vi "WristExecute.vi"(8 "error in (no error)":errorcluster) -> (0 "error out":errorcluster)   [LabVIEW 2023]
uses:
  <vilib>/Rock Robotics/WPI/ThirdParty/JAS_Junk/TrajLib/Trajectory_Library.lvlib
  WristGlobal.vi
  <vilib>/Rock Robotics/WPI/ThirdParty/REV Robotics/REVLib/SubVI/Public/SPARK Get Encoder Status Position.vi
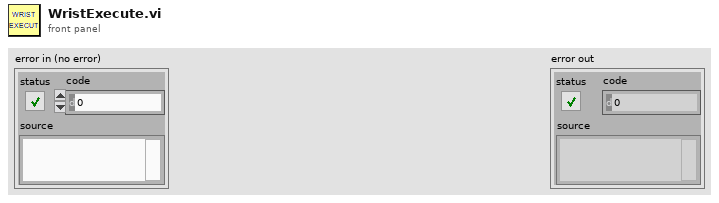
[diagram p1: front panel]
types:
  T1 = typedef "WPI_MotorControlDeviceRef.ctl" = cluster{"DeviceStatus":errorcluster, "Type":T2, "PWM":cluster{"PWM Channel":T3, "DeadBand":T4}, "CAN":cluster{"Device Number":u8, "SetOutput VI Ref":variant, "GetOutput VI Ref":variant, "Enable VI Ref":variant, "Disable VI Ref":variant, "Data":variant}, "Invert":bool, "DIO PWM":cluster{"PWM \"Enable\" Channel":T3, "DIOChannel":T5, "PWM Rate":dbl}}
  T2 = typedef "WPI_MotorControlType.ctl" = enum16{"PWM", "CAN", "DIO PWM"}
  T3 = typedef "FPGA_DIOPWMChannel.ctl" = enum8{"PWM 0", "PWM 1", "PWM 2", "PWM 3", "PWM 4", "PWM 5", "PWM 6", "PWM 7", "PWM 8", "PWM 9", "PWM MXP 0", "PWM MXP 1", "PWM MXP 2", "PWM MXP 3", "PWM MXP 4", "PWM MXP 5", "PWM MXP 6", "PWM MXP 7", "PWM MXP 8", "PWM MXP 9", "Invalid"}
  T4 = typedef "WPI_PWMDeadband.ctl" = cluster{"Name":string, "maxPositivePwm":i32, "minPositivePwm":i32, "centerPwm":i32, "maxNegativePwm":i32, "minNegativePwm":i32, "angularRange":u16}
  T5 = typedef "FPGA_DIOChannel.ctl" = enum8{"DIO 0", "DIO 1", "DIO 2", "DIO 3", "DIO 4", "DIO 5", "DIO 6", "DIO 7", "DIO 8", "DIO 9", "DIO MXP 0", "DIO MXP 1", "DIO MXP 2", "DIO MXP 3", "DIO MXP 4", "DIO MXP 5", "DIO MXP 6", "DIO MXP 7", "DIO MXP 8", "DIO MXP 9", "DIO MXP 10", "DIO MXP 11", "DIO MXP 12", "DIO MXP 13", "DIO MXP 14", "DIO MXP 15", "SPI Port CS1", "SPI Port CS2", "SPI Port CS3", "SPI Port MISO", "SPI Port MOSI", "Invalid"}
  T6 = typedef "WPI_EncoderDevRef.ctl" = cluster{"DevStatus":errorcluster, "EncoderIndex":T7, "CounterIndex":T8, "DistancePerCount":dbl, "Decoding Type":T9}
  T7 = typedef "FPGA_EncoderIdx.ctl" = enum8{"Enc 0", "Enc 1", "Enc 2", "Enc 3", "Enc 4", "Enc 5", "Enc 6", "Enc 7", "Invalid"}
  T8 = typedef "FPGA_CounterCtrSystemIndex.ctl" = enum8{"Ctr 0", "Ctr 1", "Ctr 2", "Ctr 3", "Ctr 4", "Ctr 5", "Ctr 6", "Ctr 7", "Invalid"}
  T9 = typedef "WPI_EncoderType.ctl" = enum16{"1x", "2x", "4x"}
  T10 = typedef "Trajectory_Library.lvlib/PosCtrl_Tuning_Type.ctl" = cluster{"Slope":dbl, "Offset":dbl, "Error Deadband":dbl, "At Reference Count":i32, "Negate Output":bool, "Max Allowd Position":dbl, "Min Allowd Position":dbl}
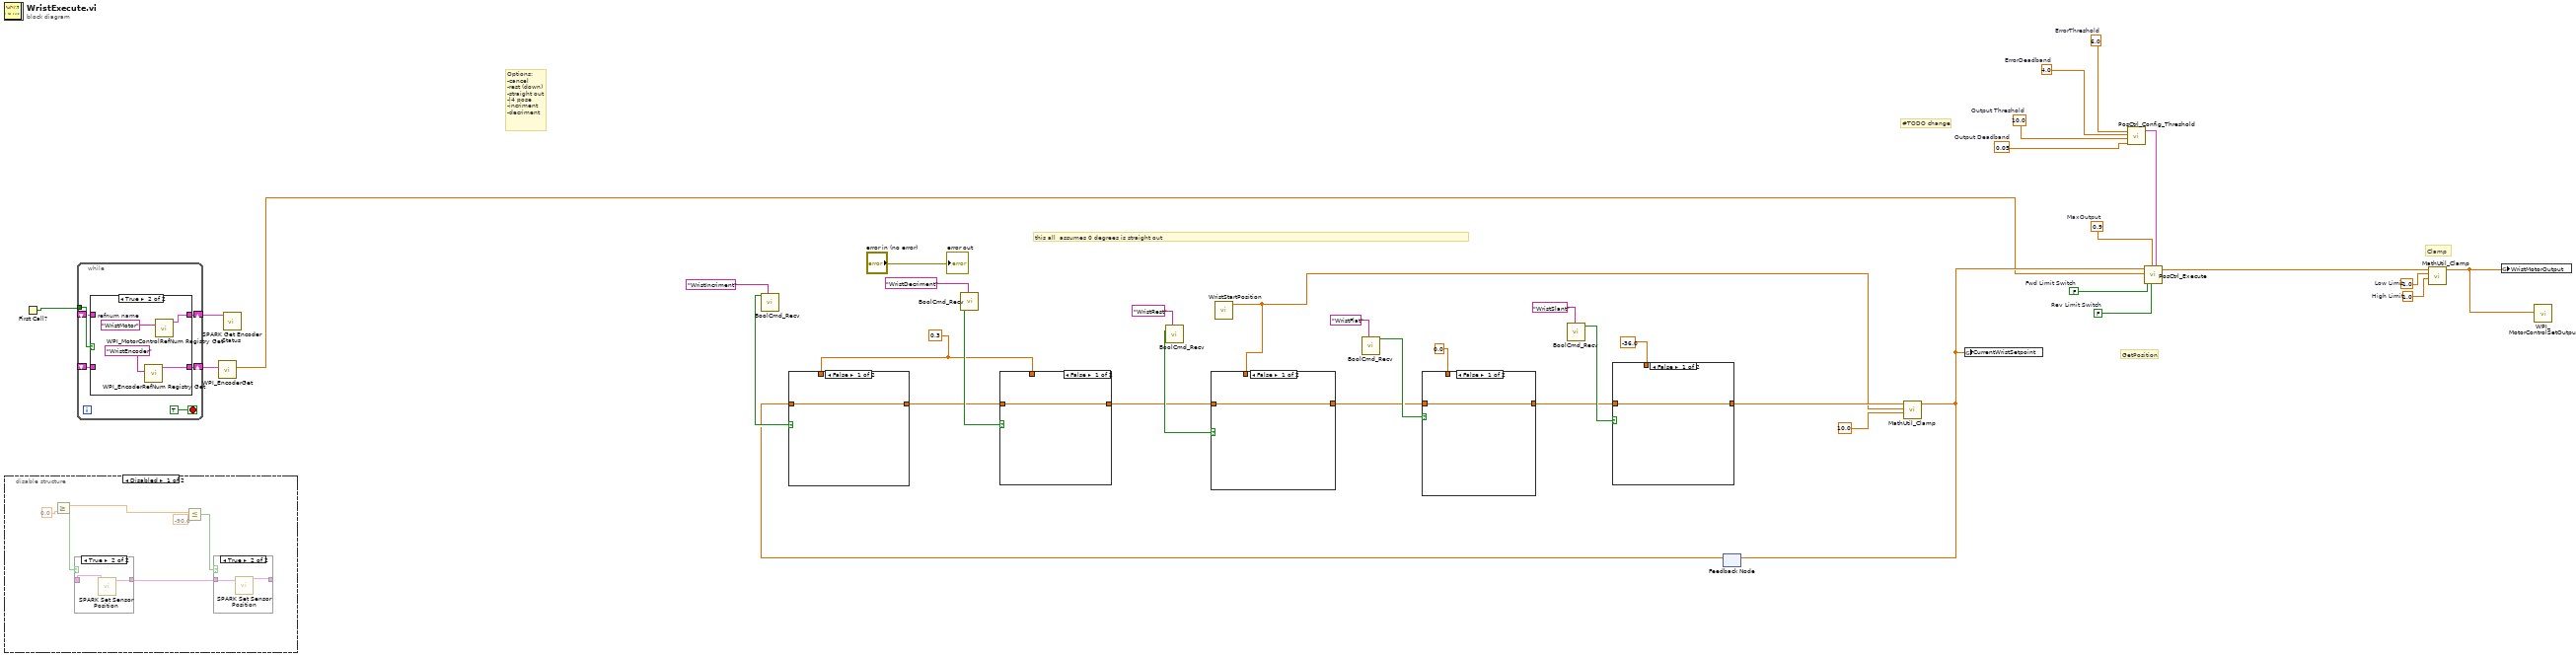
[diagram p0: block diagram]
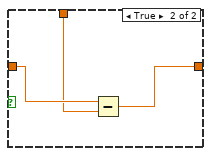
[diagram p8: hidden frame]
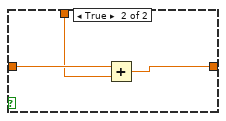
[diagram p9: hidden frame]
diagram:
  w7 = FALSE  # Fwd Limit Switch
  w8 = FALSE  # Rev Limit Switch
  w9 = 0.9  # MaxOutput
  w10 = 6.0  # ErrorThreshold
  w11 = 4.0  # ErrorDeadband
  w12 = 10.0  # Output Threshold
  w13 = 0.05  # Output Deadband
  w16 = 1.0  # High Limit
  w15 = -1.0  # Low Limit
  w22 = 0.3 ("x")
  # "GetPosition"
  # "#TODO change"
  # "Clamp"
  # "this all  assumes 0 degrees is straight out"
  # "Options:\n-cancel\n-rest (down)\n-straight out\n-l4 pose\n-incriment\n-decriment"
  n1 = disable-structure shown="Disabled" {
    frame Disabled {
      n2 = Greater Or Equal?(y=0.0) -> (x=w45:dbl, x >= y?=w44:bool)
      n3 = case shown="True" w44 {
        tunnel: _ -> [w49 w51]
        tunnel: [w49 w50] -> w40
        frame False {
        }
        frame True {
          n4 = call <vilib>:"SPARK Set Sensor Position.vi"("MotorControlDeviceRef"=w51) -> ("MotorControlDeviceRef"=w50:T1)  [unwired: 9 in, 1 out]
        }
      }
      n5 = Less Or Equal?(x=w45, y=-90.0) -> (x <= y?=w43:bool)
      n6 = case shown="True" w43 {
        tunnel: w40 -> [w46 w48]
        tunnel: [w46 w47] -> _
        frame False {
        }
        frame True {
          n7 = call <vilib>:"SPARK Set Sensor Position.vi"("MotorControlDeviceRef"=w48) -> ("MotorControlDeviceRef"=w47:T1)  [unwired: 9 in, 1 out]
        }
      }
    }
    frame Enabled {
    }
  }
  n8 = First Call?() -> (First Call?: T/F=w5:bool)
  n9 = while {
    tunnel: w5 -> [w56]
    shift-right: [w54] -> w3
    shift-left: _ -> [w53]
    shift-right: [w55] -> w4
    shift-left: _ -> [w52]
    stop <- TRUE stop-if-true
    n10 = case shown="True" w56 {
      tunnel: [w58 w61] -> w55
      tunnel: [w59 w60] -> w54
      tunnel: w53 -> [w59 _]
      tunnel: w52 -> [w58 _]
      frame False {
      }
      frame True {
        w63 = "WristMotor"  # refnum name
        n11 = call <vilib>:"WPI_EncoderRefNum Registry Get.vi"("refnum name"="WristEncoder") -> ("EncoderDevRef"=w61:T6)  [unwired: 9 in, 1 out]
        n12 = call <vilib>:"WPI_MotorControlRefNum Registry Get.vi"("refnum name"=w63) -> ("MotorControlDevRef"=w60:T1)  [unwired: 9 in, 1 out]
      }
    }
  }
  n13 = call <vilib>:"WPI_EncoderGet.vi"("EncoderDevRef"=w4) -> ("Distance"=w1:dbl)  [unwired: 5 in, 5 out]
  n14 = call-poly <vilib>:"SPARK Get Encoder Status.vi"("MotorControlDevRef in"=w3) -> ()  [unwired: 7 in, 4 out]
  n15 = call <vilib>:"BoolCmd_Recv.vi"("Command Name"="WristIncriment") -> ("New Request"=w35:bool)  [unwired: 9 in, 1 out]
  n16 = call <vilib>:"BoolCmd_Recv.vi"("Command Name"="WristDecriment") -> ("New Request"=w33:bool)  [unwired: 9 in, 1 out]
  n17 = call <vilib>:"BoolCmd_Recv.vi"("Command Name"="WristRest") -> ("New Request"=w37:bool)  [unwired: 9 in, 1 out]
  n18 = call "WristStartPosition.vi"() -> ("Numeric"=w17:dbl)  [unwired: 10 in, 1 out]
  n19 = call <vilib>:"BoolCmd_Recv.vi"("Command Name"="WristFlat") -> ("New Request"=w31:bool)  [unwired: 9 in, 1 out]
  n20 = call <vilib>:"BoolCmd_Recv.vi"("Command Name"="WristSlant") -> ("New Request"=w29:bool)  [unwired: 9 in, 1 out]
  n21 = feedback #1() -> (w28:dbl)  [unwired: 1 in]
  n22 = case shown="False" w35 {
    tunnel: w28 -> [w64 w66]
    tunnel: [w64 w67] -> w27
    tunnel: w22 -> [_ w65]
    frame False {
    }
    frame True {
      n23 = Add(x=w66, y=w65) -> (x+y=w67:dbl)
    }
  }
  n24 = case shown="False" w33 {
    tunnel: w27 -> [w68 w70]
    tunnel: [w68 w71] -> w26
    tunnel: w22 -> [_ w69]
    frame False {
    }
    frame True {
      n25 = Subtract(x=w70, y=w69) -> (x-y=w71:dbl)
    }
  }
  n26 = case shown="False" w37 {
    tunnel: w26 -> [w72 _]
    tunnel: [w72 w73] -> w25
    tunnel: w17 -> [_ w73]
    frame False {
    }
    frame True {
    }
  }
  n27 = case shown="False" w31 {
    tunnel: w25 -> [w74 _]
    tunnel: [w74 w75] -> w24
    tunnel: 0.0 ("Result") -> [_ w75]
    frame False {
    }
    frame True {
    }
  }
  n28 = case shown="False" w29 {
    tunnel: w24 -> [w76 _]
    tunnel: [w76 w77] -> w23
    tunnel: -36.0 ("Result") -> [_ w77]
    frame False {
    }
    frame True {
    }
  }
  n29 = call <vilib>:"MathUtil_Clamp.vi"("High Limit"=10.0, "Low Limit"=w17, "Value"=w23) -> ("Result"=w6:dbl)  [unwired: 8 in]
  n30 = feedback-in #1(w6) -> ()
  n31 = global write "WristGlobal.vi" "CurrentWristSetpoint"(w6) -> ()
  n32 = call <vilib>:"PosCtrl_Config_Threshold.vi"("Output Deadband"=w13, "Output Threshold"=w12, "ErrorDeadband"=w11, "ErrorThreshold"=w10) -> ("PosCtrl_Config_Params"=w18:T10)  [unwired: 7 in]
  n33 = call <vilib>:"PosCtrl_Execute.vi"("PosCtrl_Config_Params"=w18, "MaxOutput"=w9, "Rev Limit Switch"=w8, "Fwd Limit Switch"=w7, "CurrentPosition"=w1, "TargetPosition"=w6) -> ("Output"=w14:dbl)  [unwired: 3 in, 2 out]
  n34 = call <vilib>:"MathUtil_Clamp.vi"("High Limit"=w16, "Low Limit"=w15, "Value"=w14) -> ("Result"=w2:dbl)  [unwired: 8 in]
  n35 = global write "WristGlobal.vi" "WristMotorOutput"(w2) -> ()
  n36 = call <vilib>:"WPI_MotorControlSetOutput.vi"("Output"=w2) -> ()  [unwired: 8 in, 3 out]
  "error out" <- "error in (no error)"
